vi "Control Panel.vi"(8 "error in (no error)":errorcluster, 11 "Fake Pulse Generator in":refnum<class "Pulse Generator.lvclass">) -> (0 "error out":errorcluster, 3 "Fake Pulse Generator out":refnum<class "Pulse Generator.lvclass">)   [LabVIEW 2017, in "Pulse Generator.lvclass"]
uses:
  Pulse Generator.lvclass
  Pulse Generator.lvclass/Pulse Generator.ctl
  Utility Classes/Scannable/Scannable.lvclass
panel:
  in  "Ch1/Ch2 Toggle":bool
  in  "Width/Duty\nUP/DOWN Ch2":bool
  in  "Width/Duty\nUP/DOWN Ch1":bool
  in  "Clear Error":bool
  out "Ready when \nblinking":bool
  in  "Copy actual to set":bool
  out "Pulse Mode":enum16{"Pulses", "Pattern"}(ring)
  out "Arming (Trigger) Source":T1(ring)
  in  "Populate fields with member data":bool
  out "Strobe Pattern":string
  in  "Strobe Pattern Set":string
  out "StrobeDataBuffer":digitalwaveform(graph)
  in  "Enable/disable":bool
  in  "Modes (changes immediately)":T2(radio)
  in  "BitPeriodSet":dbl[unit]
  out "BitPeriod":dbl[unit]
  out "Ch2Pattern":string
  in  "Ch2Pattern Set":string
  out "Ch1Pattern":string
  in  "Set Patterns":bool
  in  "Ch1Pattern Set":string
  in  "Ch2Duty (%) Set":dbl=10.0
  in  "Ch1Duty (%) Set":dbl=10.0
  in  "Ch1Delay Set":dbl[unit]
  in  "Ch2Delay Set":dbl[unit]
  in  "stop":bool
  out "Ch1DataBuffer":digitalwaveform(graph)
  out "Ch2DataBuffer":digitalwaveform(graph)
  in  "Ch2 Sync":bool
  in  "Ch1 Sync":bool
  in  "Ch2 Toggle":bool
  in  "Ch1 NOT Toggle":bool
  in  "Ch1 Toggle":bool
  in  "Ch2 NOT Toggle":bool
  in  "OverallPeriodSet":dbl[unit]
  in  "Ch2WidthSet":dbl[unit]=1e-09
  in  "Ch1WidthSet":dbl[unit]=1e-09
  in  "Ch2LowSet":dbl[unit]
  in  "Ch2HighSet":dbl[unit]
  in  "Ch1LowSet":dbl[unit]
  in  "Ch1HighSet":dbl[unit]
  in  "OverallFreqSet":dbl[unit]
  in  "Read to Control":bool
  in  "Set":bool
  out "Ch2Duty (%)":dbl
  out "Ch1Duty (%)":dbl
  out "Ch1Delay":dbl[unit]
  out "Ch2Delay":dbl[unit]
  out "Ch1Low":dbl[unit]
  out "Ch1High":dbl[unit]
  out "Ch2Width":dbl[unit]
  out "Ch1Width":dbl[unit]
  out "OverallPeriod":dbl[unit]
  out "Ch2Low":dbl[unit]
  out "Ch2High":dbl[unit]
  in  "Read":bool
  out "OverallFreq":dbl[unit]
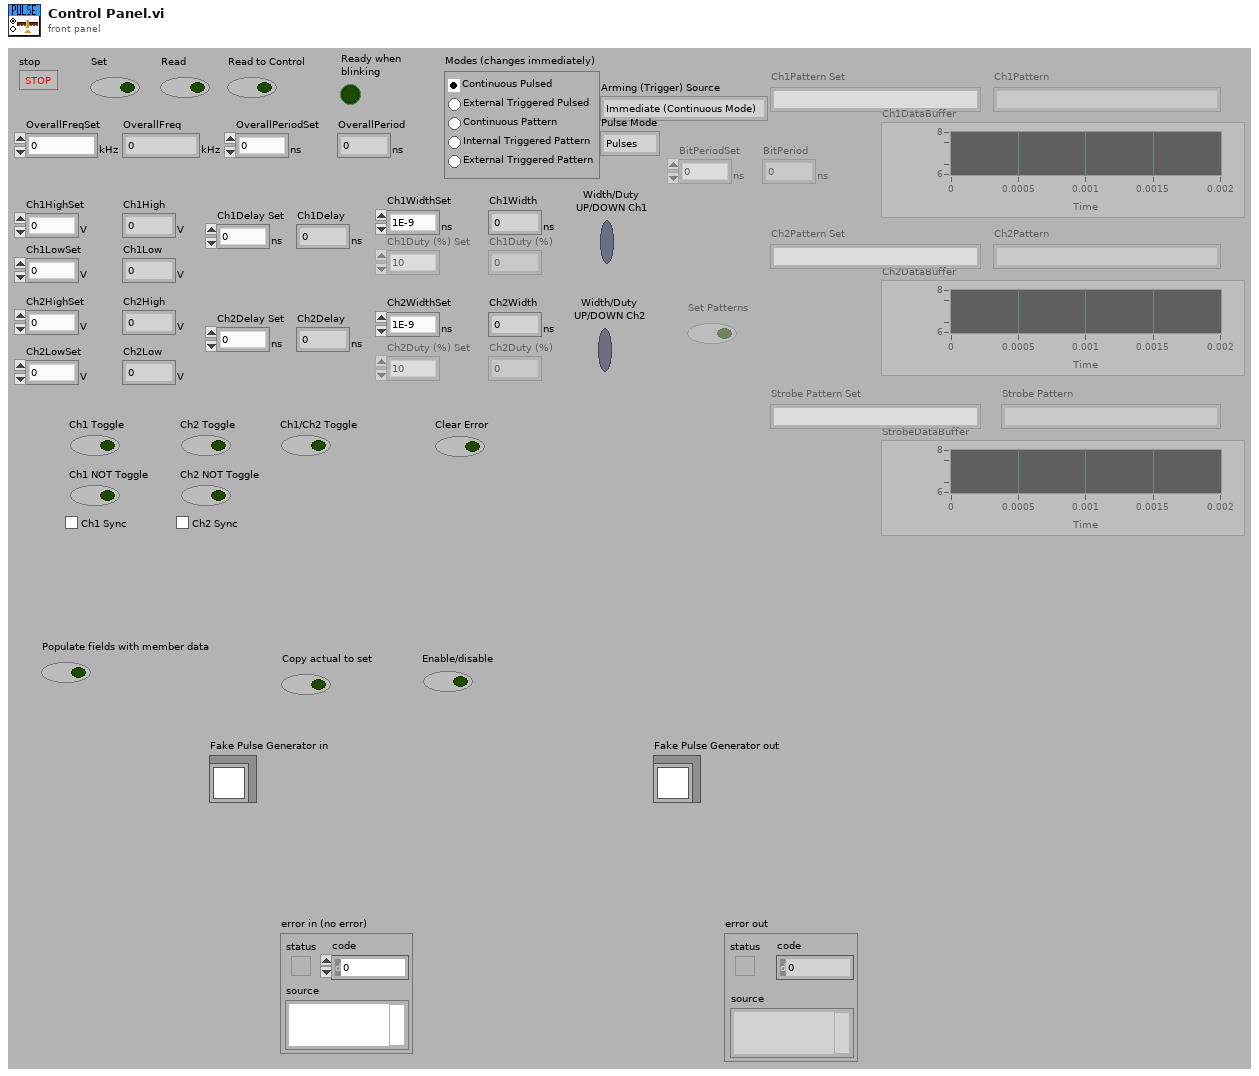
[diagram p1: front panel]
types:
  T1 = enum16{"Immediate (Continuous Mode)", "Internal PLL", "External", "Manual"}
  T2 = enum32{"Continuous Pulsed", "Continuous Pattern", "Internal Triggered Pattern", "External Triggered Pulsed", "External Triggered Pattern", "Other"}
  T3 = enum16{"Internal Oscillator", "Internal PLL", "External Clock "}
  T4 = enum16{"Internal Oscillator", "Internal PLL", "Clock Input"}
  T5 = enum16{"Channel All ", "Channel 1", "Channel 2", "Channel 3", "Channels Combined"}
  T6 = cluster{"1 High":dbl[unit], "1 Low":dbl[unit], "2 High":dbl[unit], "2 Low":dbl[unit]}
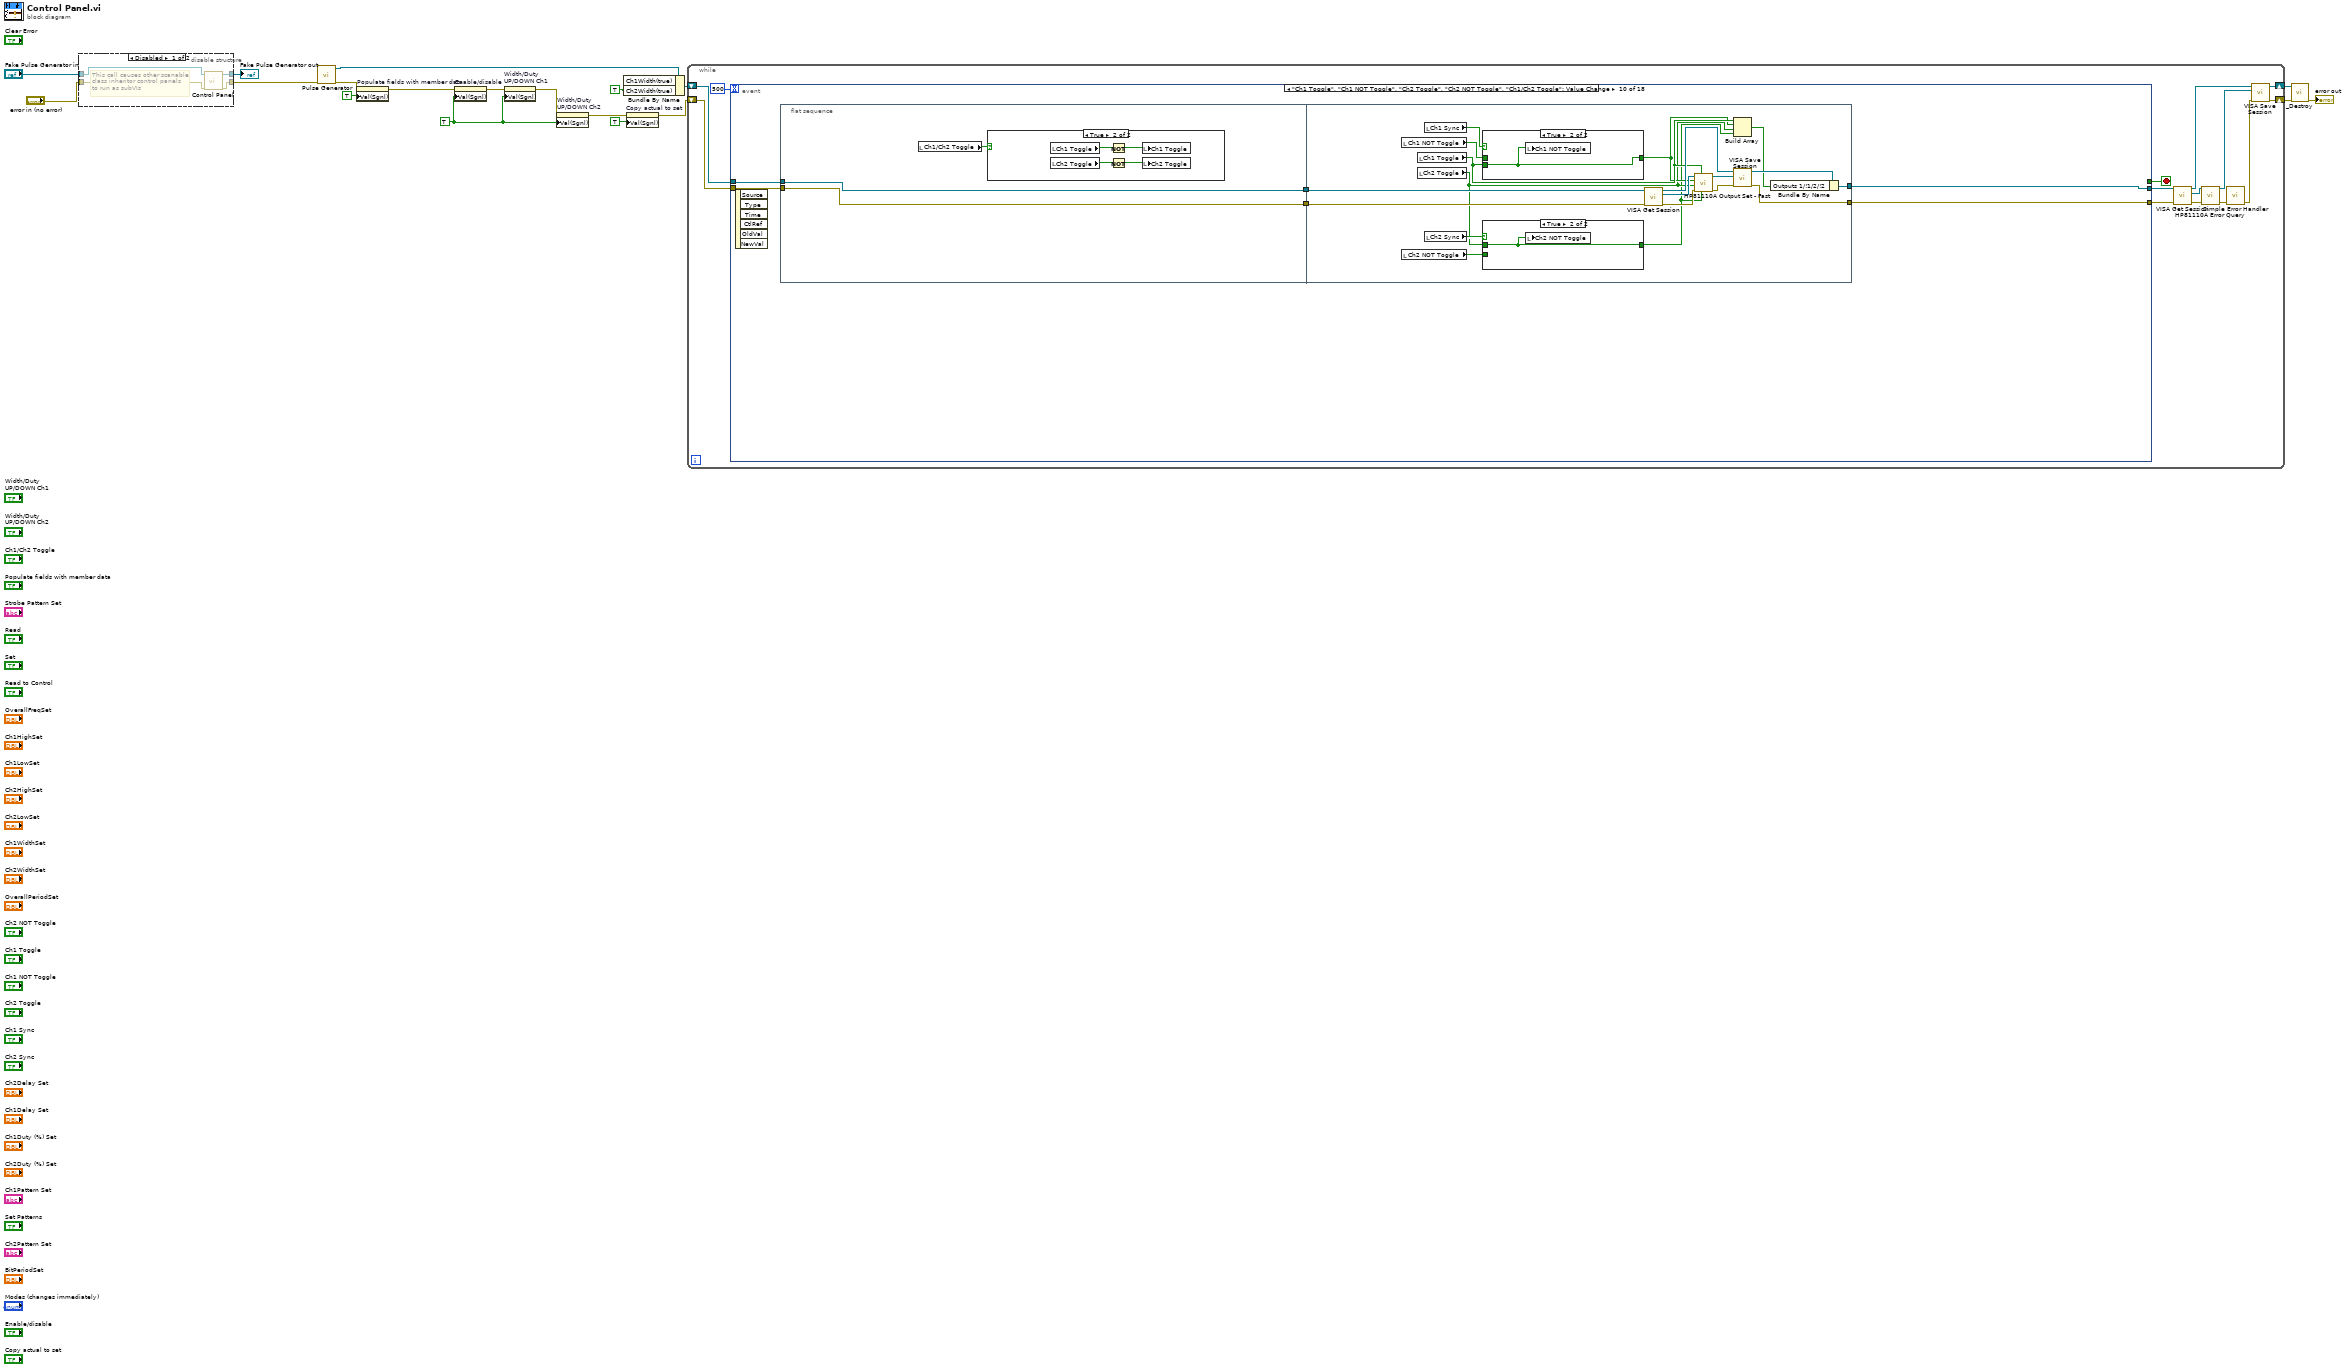
[diagram p0: block diagram]
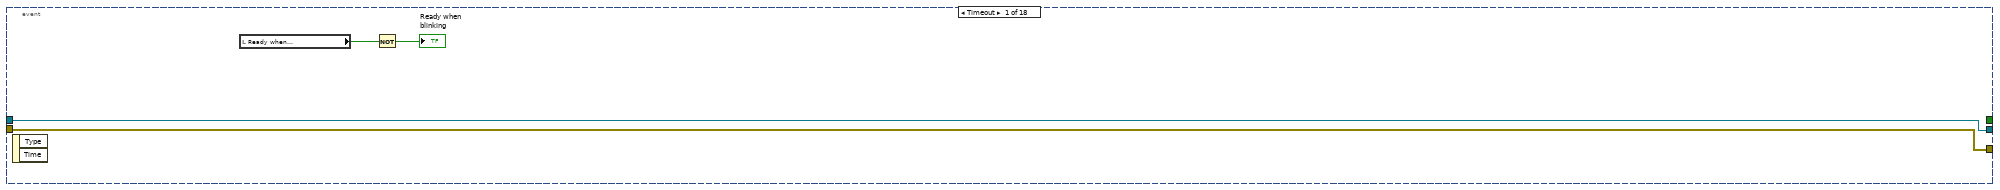
[diagram p3: hidden frame]
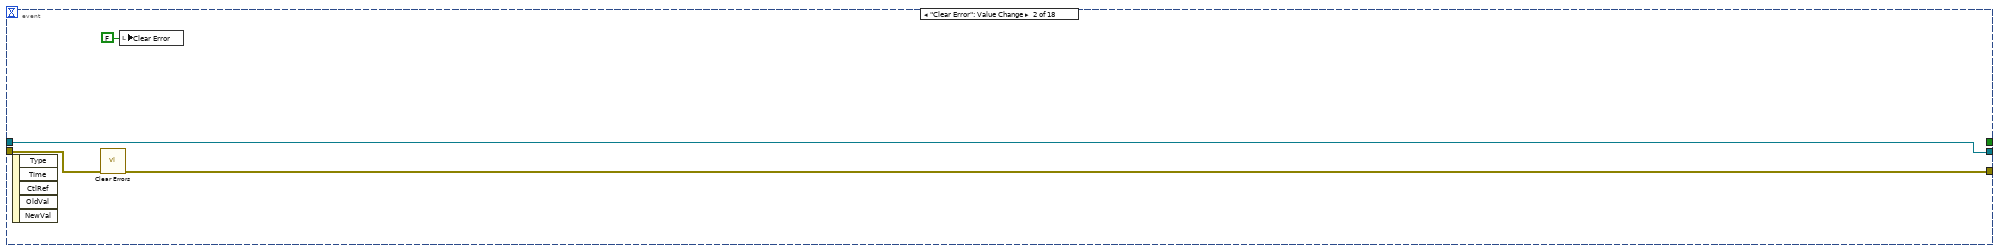
[diagram p4: hidden frame]
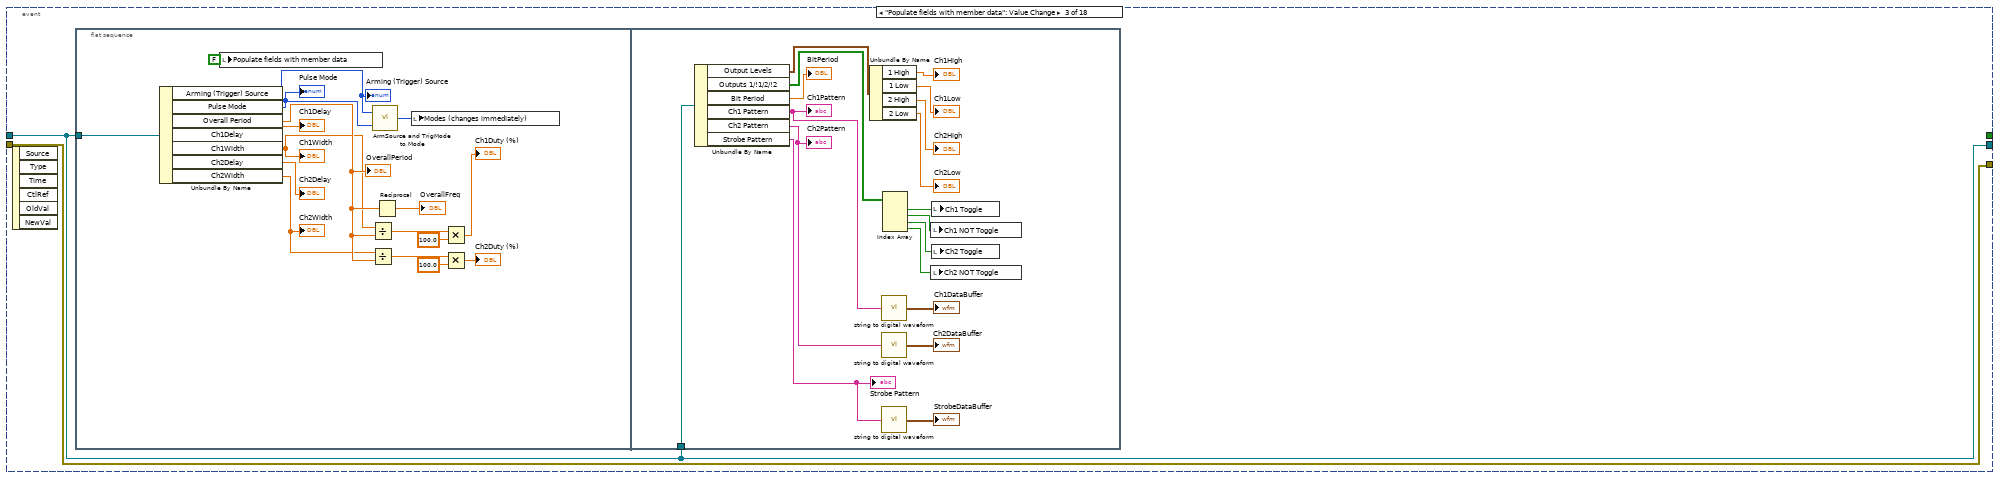
[diagram p5: hidden frame]
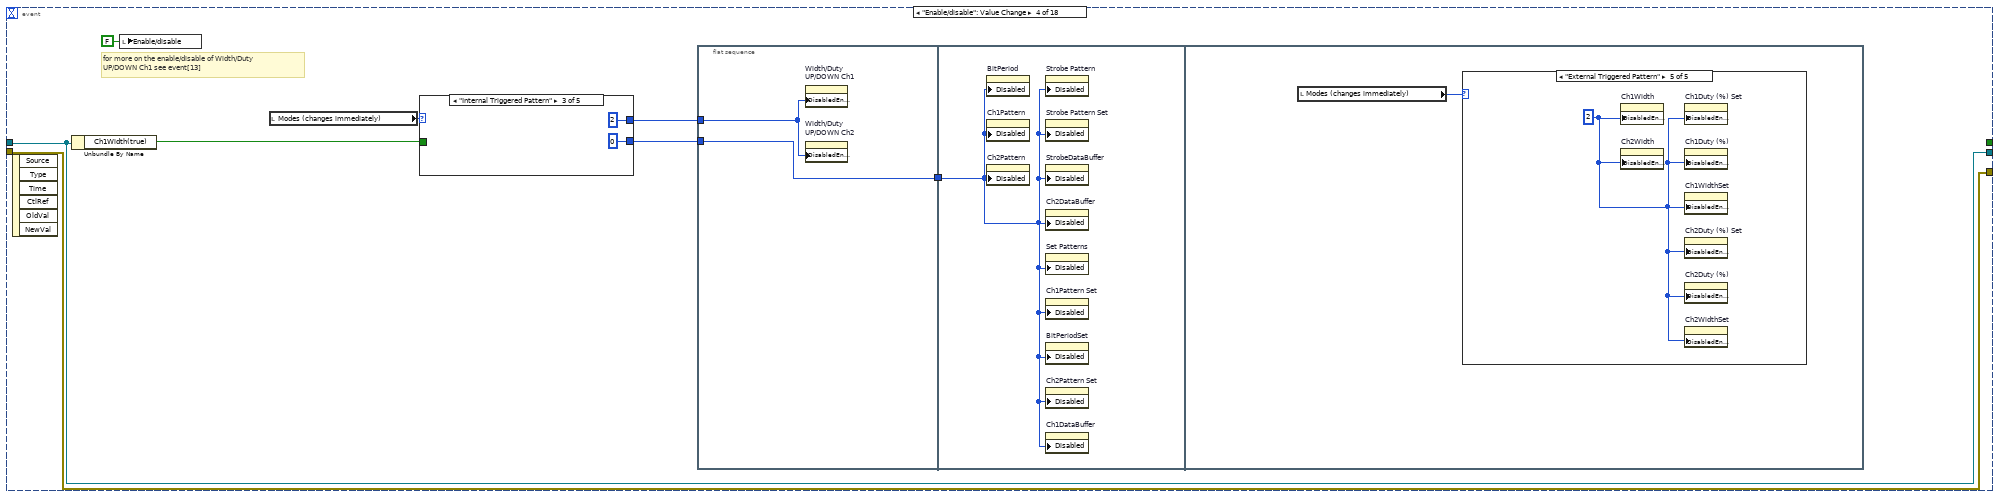
[diagram p6: hidden frame]
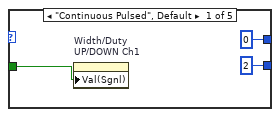
[diagram p7: hidden frame]
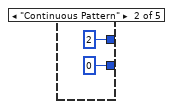
[diagram p8: hidden frame]
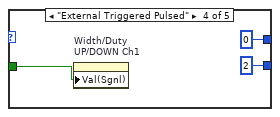
[diagram p9: hidden frame]
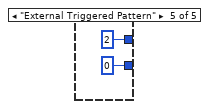
[diagram p10: hidden frame]
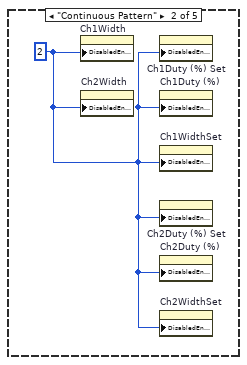
[diagram p12: hidden frame]
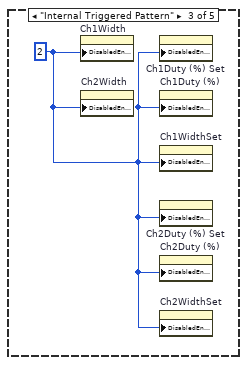
[diagram p13: hidden frame]
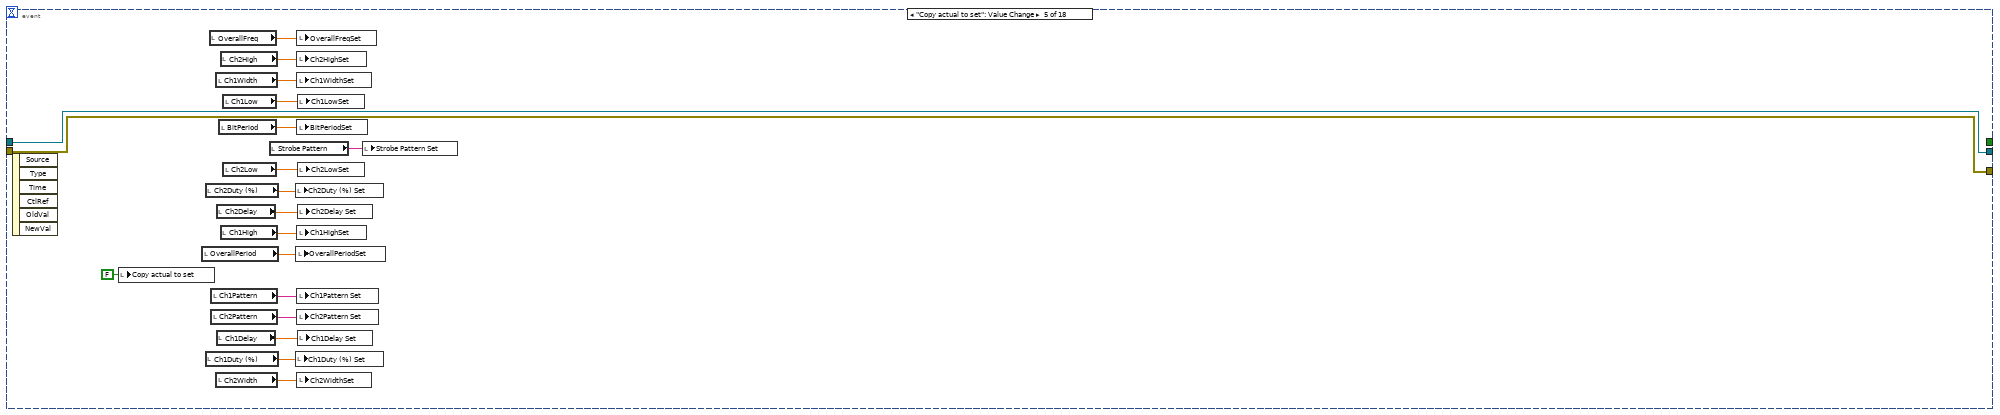
[diagram p15: hidden frame]
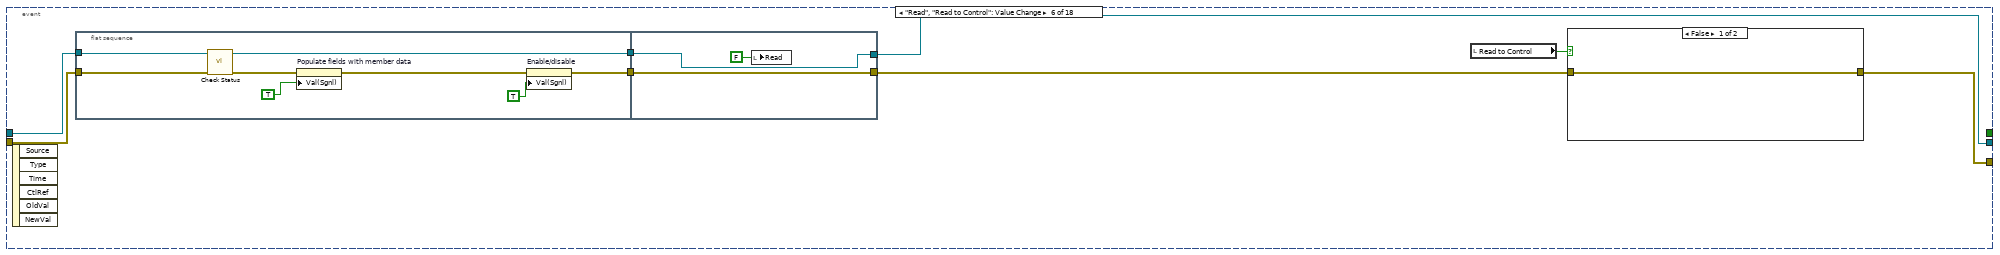
[diagram p16: hidden frame]
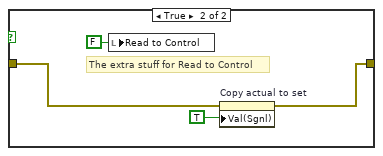
[diagram p17: hidden frame]
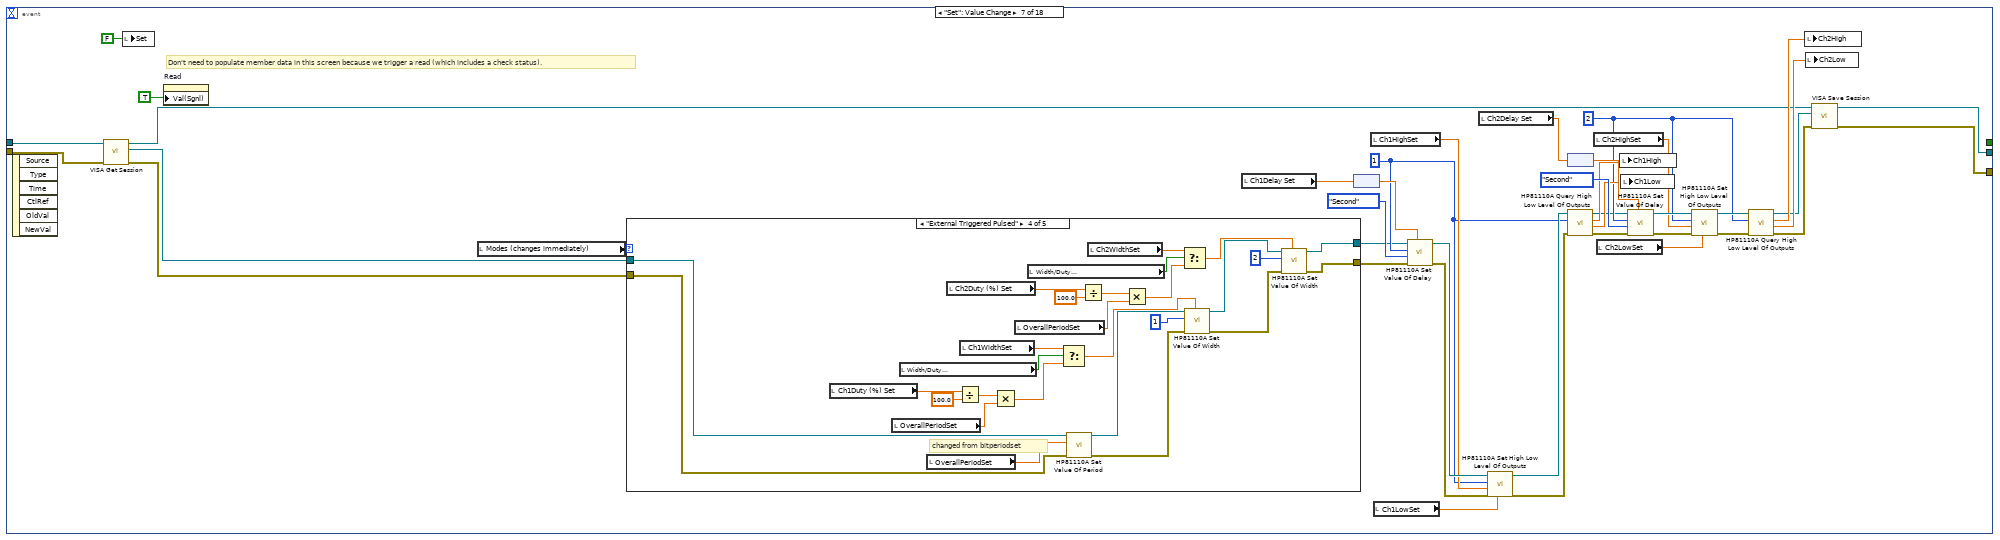
[diagram p18: hidden frame]
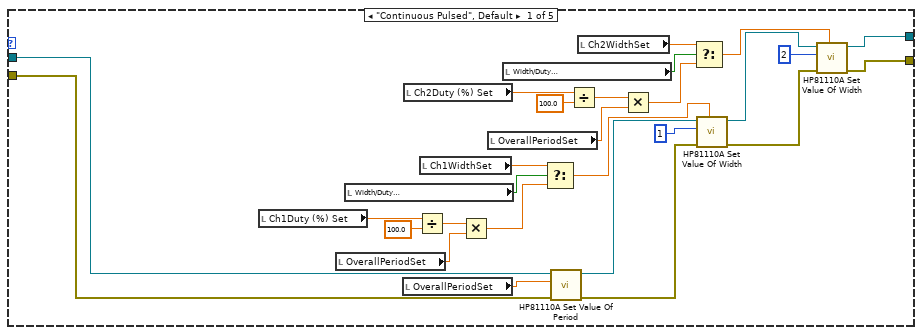
[diagram p19: hidden frame]
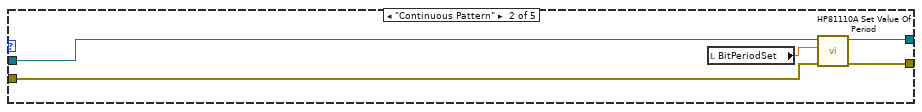
[diagram p20: hidden frame]
diagram:
  w1 = TRUE
  w4 = TRUE ("Value (Signaling)")
  n1 = disable-structure shown="Disabled" {
    disable-tunnel: [w23 w25] -> w19
    disable-tunnel: "error in (no error)" -> [w22 w24]
    disable-tunnel: "Fake Pulse Generator in" -> [w21 w25]
    disable-tunnel: [w20 w24] -> w11
    frame Disabled {
      # "This call causes other scanable\nclass inheritor control panels\nto run as subVIs"
      n2 = call-parent "Control Panel.vi"("error in (no error)"=w22, "Instrument in"=w21) -> ("error out"=w20:errorcluster, "Instrument out"=w23:refnum<class "Pulse Generator.lvclass">)  [unwired: 8 out]
    }
    frame Enabled {
    }
  }
  "Fake Pulse Generator out" <- w19
  n3 = call "Pulse Generator.vi"("error in (no error)"=w11) -> ("error out"=w12:errorcluster, "Pulse Generator out"=w3:refnum<class "Pulse Generator.lvclass">)  [unwired: 9 out]
  n4 = property on="Populate fields with member data" class="Bool (strict)"(error in=w12, "Val(Sgnl)"=TRUE ("Value (Signaling)")) -> (error out=w9:errorcluster)  [unwired: 1 in, 1 out]
  n5 = property on="Enable/disable" class="Bool (strict)"(error in=w9, "Val(Sgnl)"=w4) -> (error out=w7:errorcluster)  [unwired: 1 in, 1 out]
  n6 = property on="Width/Duty\nUP/DOWN Ch1" class="Bool (strict)"(error in=w7, "Val(Sgnl)"=w4) -> (error out=w5:errorcluster)  [unwired: 1 in, 1 out]
  n7 = property on="Width/Duty\nUP/DOWN Ch2" class="Bool (strict)"(error in=w5, "Val(Sgnl)"=w4) -> (error out=w6:errorcluster)  [unwired: 1 in, 1 out]
  n8 = Bundle By Name(cluster=w3, "Ch1Width(true)"=w1, "Ch2Width(true)"=w1) -> (w2:refnum<class "Pulse Generator.lvclass">)
  n9 = property on="Copy actual to set" class="Bool (strict)"(error in=w6, "Val(Sgnl)"=TRUE ("Value (Signaling)")) -> (error out=w8:errorcluster)  [unwired: 1 in, 1 out]
  n10 = while {
    shift-right: [w32] -> w16
    shift-left: w2 -> [w37]
    shift-right: [w27] -> w15
    shift-left: w8 -> [w36]
    stop <- w39 stop-if-true
    n11 = event shown="[9] \"Ch1 Toggle\", \"Ch1 NOT Toggle\", \"Ch2 Toggle\", \"Ch2 NOT Toggle\", \"Ch1/Ch2 Toggle\": Value Change" {
      selector: _ -> [_ _ _ _ _ _ _ _ _ _ _ _ _ _ _ _ _ _]
      dyn-events: _ -> [_ _ _ _ _ _ _ _ _ _ _ _ _ _ _ _ _ _]
      timeout: 500 -> [_ _ _ _ _ _ _ _ _ _ _ _ _ _ _ _ _ _]
      tunnel: [_ _ _ _ _ _ _ _ _ _ _ _ "stop" _ _ _ _ _] -> w39
      tunnel: w36 -> [w42 w47 w49 w91 w113 w138 w161 w273 w311 w327 w362 w385 w398 w418 w420 w430 w440 w446]
      tunnel: [w42 w45 w49 w91 w113 w134 w157 w269 w305 w326 w362 w385 w398 w418 w420 w430 w440 w446] -> w30
      tunnel: w37 -> [w43 w46 w48 w86 w114 w137 w163 w275 w312 w328 w363 w386 w397 w405 w419 w429 w439 w447]
      tunnel: [w43 w46 w48 w86 w114 w136 w158 w270 w307 w325 w363 w386 w397 w404 w419 w429 w439 w447] -> w31
      event Timeout {
        n12 = event-data() -> ()  [unwired: 3 out]
        n13 = local read "Ready when \nblinking"() -> (w41:bool)
        n14 = Not(x=w41) -> (.not. x?=→"Ready when \nblinking":bool)
      }
      event "Clear Error": Value Change {
        n15 = event-data() -> ()  [unwired: 6 out]
        n16 = call <vilib>:"Clear Errors.vi"("error in (no error)"=w47) -> ("error out"=w45:errorcluster)  [unwired: 5 in, 1 out]
        n17 = local write "Clear Error"(FALSE ("Clear Error")) -> ()
      }
      event "Populate fields with member data": Value Change {
        n18 = event-data() -> ()  [unwired: 7 out]
        n19 = flat-sequence {
          tunnel: w48 -> [w56]
          tunnel: w48 -> [w67]
          frame #0 {
            n20 = Unbundle By Name(w56) -> ("Arming (Trigger) Source"=w59:u16, "Pulse Mode"=w58:u16, "Overall Period"=w62:dbl[unit], "Ch1Delay"=→"Ch1Delay":dbl[unit], "Ch1Width"=w61:dbl[unit], "Ch2Delay"=→"Ch2Delay":dbl[unit], "Ch2Width"=w60:dbl[unit])
            "OverallPeriod" <- w62
            "Ch1Width" <- w61
            "Ch2Width" <- w60
            "Arming (Trigger) Source" <- w59
            "Pulse Mode" <- w58
            n21 = local write "Populate fields with member data"(FALSE ("Populate fields with member data")) -> ()
            n22 = Divide(x=w61, y=w62) -> (x/y=w53:dbl)
            n23 = Divide(x=w60, y=w62) -> (x/y=w51:dbl)
            n24 = call "ArmSource and TrigMode to Mode.vi"("Pulse Mode"=w58, "Arming (Trigger) Source (0:Internal PLL)"=w59) -> ("Modes (changes immediately)"=w57:T2)
            n25 = Reciprocal(x=w62) -> (1/x=→"OverallFreq":dbl[unit])
            n26 = local write "Modes (changes immediately)"(w57) -> ()
            n27 = Multiply(x=w53, y=100.0) -> (x*y=→"Ch1Duty (%)":dbl)
            n28 = Multiply(x=w51, y=100.0) -> (x*y=→"Ch2Duty (%)":dbl)
          }
          frame #1 {
            n29 = Unbundle By Name(w67) -> ("Output Levels"=w79:T6, "Outputs 1/!1/2/!2"=w80:bool[], "Bit Period"=→"BitPeriod":dbl[unit], "Ch1 Pattern"=w82:string, "Ch2 Pattern"=w83:string, "Strobe Pattern"=w84:string)
            "Ch1Pattern" <- w82
            "Ch2Pattern" <- w83
            "Strobe Pattern" <- w84
            n30 = Unbundle By Name(w79) -> ("1 High"=→"Ch1High":dbl[unit], "1 Low"=→"Ch1Low":dbl[unit], "2 High"=→"Ch2High":dbl[unit], "2 Low"=→"Ch2Low":dbl[unit])
            n31 = call "string to digital waveform.vi"("String"=w82) -> ("digital waveform"=→"Ch1DataBuffer":digitalwaveform)
            n32 = call "string to digital waveform.vi"("String"=w83) -> ("digital waveform"=→"Ch2DataBuffer":digitalwaveform)
            n33 = call "string to digital waveform.vi"("String"=w84) -> ("digital waveform"=→"StrobeDataBuffer":digitalwaveform)
            n34 = Index Array(array=w80) -> (element #1=w75:bool, element #2=w76:bool, element #3=w77:bool, element #4=w78:bool)  [unwired: 4 in]
            n35 = local write "Ch1 NOT Toggle"(w76) -> ()
            n36 = local write "Ch2 NOT Toggle"(w78) -> ()
            n37 = local write "Ch1 Toggle"(w75) -> ()
            n38 = local write "Ch2 Toggle"(w77) -> ()
          }
        }
      }
      event "Enable/disable": Value Change {
        # "for more on the enable/disable of Width/Duty\nUP/DOWN Ch1 see event[13]"
        n39 = event-data() -> ()  [unwired: 7 out]
        n40 = Unbundle By Name(w86) -> ("Ch1Width(true)"=w85:bool)
        n41 = local write "Enable/disable"(FALSE ("Enable/disable")) -> ()
        n42 = local read "Modes (changes immediately)"() -> (w89:T2)
        n43 = case shown="\"Internal Triggered Pattern\"" w89 {
          tunnel: [2 0 0 2 0] -> w87
          tunnel: [0 2 2 0 2] -> w88
          tunnel: w85 -> [w93 _ _ w100 _]
          frame "Continuous Pulsed", Default {
            n44 = property on="Width/Duty\nUP/DOWN Ch1" class="Bool (strict)"("Val(Sgnl)"=w93) -> ()  [unwired: 2 in, 2 out]
          }
          frame "Continuous Pattern" {
          }
          frame "Internal Triggered Pattern" {
          }
          frame "External Triggered Pulsed" {
            n45 = property on="Width/Duty\nUP/DOWN Ch1" class="Bool (strict)"("Val(Sgnl)"=w100) -> ()  [unwired: 2 in, 2 out]
          }
          frame "External Triggered Pattern" {
          }
        }
        n46 = flat-sequence {
          tunnel: [w106] -> w90
          tunnel: w88 -> [w105]
          tunnel: w87 -> [w106]
          tunnel: w90 -> [w107]
          frame #0 {
            n47 = property on="Width/Duty\nUP/DOWN Ch1" class="Bool (strict)"("DisabledEnum"=w105) -> ()  [unwired: 2 in, 2 out]
            n48 = property on="Width/Duty\nUP/DOWN Ch2" class="Bool (strict)"("DisabledEnum"=w105) -> ()  [unwired: 2 in, 2 out]
          }
          frame #1 {
            n49 = property on="BitPeriod" class="DigNum (strict)"("Disabled"=w107) -> ()  [unwired: 2 in, 2 out]
            n50 = property on="Ch1Pattern" class="Str"("Disabled"=w107) -> ()  [unwired: 2 in, 2 out]
            n51 = property on="Ch2Pattern" class="Str"("Disabled"=w107) -> ()  [unwired: 2 in, 2 out]
            n52 = property on="Strobe Pattern" class="Str"("Disabled"=w107) -> ()  [unwired: 2 in, 2 out]
            n53 = property on="Strobe Pattern Set" class="Str"("Disabled"=w107) -> ()  [unwired: 2 in, 2 out]
            n54 = property on="StrobeDataBuffer" class="DigitalGraph (strict)"("Disabled"=w107) -> ()  [unwired: 2 in, 2 out]
            n55 = property on="Ch2DataBuffer" class="DigitalGraph (strict)"("Disabled"=w107) -> ()  [unwired: 2 in, 2 out]
            n56 = property on="Set Patterns" class="Bool (strict)"("Disabled"=w107) -> ()  [unwired: 2 in, 2 out]
            n57 = property on="Ch1Pattern Set" class="Str"("Disabled"=w107) -> ()  [unwired: 2 in, 2 out]
            n58 = property on="BitPeriodSet" class="DigNum (strict)"("Disabled"=w107) -> ()  [unwired: 2 in, 2 out]
            n59 = property on="Ch2Pattern Set" class="Str"("Disabled"=w107) -> ()  [unwired: 2 in, 2 out]
            n60 = property on="Ch1DataBuffer" class="DigitalGraph (strict)"("Disabled"=w107) -> ()  [unwired: 2 in, 2 out]
          }
          frame #2 {
            n61 = local read "Modes (changes immediately)"() -> (w108:T2)
            n62 = case shown="\"External Triggered Pattern\"" w108 {
              frame "Continuous Pulsed", Default {
              }
              frame "Continuous Pattern" {
                w109 = 2
                n63 = property on="Ch1Width" class="DigNum (strict)"("DisabledEnum"=w109) -> ()  [unwired: 2 in, 2 out]
                n64 = property on="Ch2Width" class="DigNum (strict)"("DisabledEnum"=w109) -> ()  [unwired: 2 in, 2 out]
                n65 = property on="Ch1Duty (%) Set" class="DigNum (strict)"("DisabledEnum"=w109) -> ()  [unwired: 2 in, 2 out]
                n66 = property on="Ch1Duty (%)" class="DigNum (strict)"("DisabledEnum"=w109) -> ()  [unwired: 2 in, 2 out]
                n67 = property on="Ch1WidthSet" class="DigNum (strict)"("DisabledEnum"=w109) -> ()  [unwired: 2 in, 2 out]
                n68 = property on="Ch2Duty (%) Set" class="DigNum (strict)"("DisabledEnum"=w109) -> ()  [unwired: 2 in, 2 out]
                n69 = property on="Ch2Duty (%)" class="DigNum (strict)"("DisabledEnum"=w109) -> ()  [unwired: 2 in, 2 out]
                n70 = property on="Ch2WidthSet" class="DigNum (strict)"("DisabledEnum"=w109) -> ()  [unwired: 2 in, 2 out]
              }
              frame "Internal Triggered Pattern" {
                w110 = 2
                n71 = property on="Ch1Width" class="DigNum (strict)"("DisabledEnum"=w110) -> ()  [unwired: 2 in, 2 out]
                n72 = property on="Ch2Width" class="DigNum (strict)"("DisabledEnum"=w110) -> ()  [unwired: 2 in, 2 out]
                n73 = property on="Ch1Duty (%) Set" class="DigNum (strict)"("DisabledEnum"=w110) -> ()  [unwired: 2 in, 2 out]
                n74 = property on="Ch1Duty (%)" class="DigNum (strict)"("DisabledEnum"=w110) -> ()  [unwired: 2 in, 2 out]
                n75 = property on="Ch1WidthSet" class="DigNum (strict)"("DisabledEnum"=w110) -> ()  [unwired: 2 in, 2 out]
                n76 = property on="Ch2Duty (%) Set" class="DigNum (strict)"("DisabledEnum"=w110) -> ()  [unwired: 2 in, 2 out]
                n77 = property on="Ch2Duty (%)" class="DigNum (strict)"("DisabledEnum"=w110) -> ()  [unwired: 2 in, 2 out]
                n78 = property on="Ch2WidthSet" class="DigNum (strict)"("DisabledEnum"=w110) -> ()  [unwired: 2 in, 2 out]
              }
              frame "External Triggered Pulsed" {
              }
              frame "External Triggered Pattern" {
                w111 = 2
                n79 = property on="Ch1Width" class="DigNum (strict)"("DisabledEnum"=w111) -> ()  [unwired: 2 in, 2 out]
                n80 = property on="Ch2Width" class="DigNum (strict)"("DisabledEnum"=w111) -> ()  [unwired: 2 in, 2 out]
                n81 = property on="Ch1Duty (%) Set" class="DigNum (strict)"("DisabledEnum"=w111) -> ()  [unwired: 2 in, 2 out]
                n82 = property on="Ch1Duty (%)" class="DigNum (strict)"("DisabledEnum"=w111) -> ()  [unwired: 2 in, 2 out]
                n83 = property on="Ch1WidthSet" class="DigNum (strict)"("DisabledEnum"=w111) -> ()  [unwired: 2 in, 2 out]
                n84 = property on="Ch2Duty (%) Set" class="DigNum (strict)"("DisabledEnum"=w111) -> ()  [unwired: 2 in, 2 out]
                n85 = property on="Ch2Duty (%)" class="DigNum (strict)"("DisabledEnum"=w111) -> ()  [unwired: 2 in, 2 out]
                n86 = property on="Ch2WidthSet" class="DigNum (strict)"("DisabledEnum"=w111) -> ()  [unwired: 2 in, 2 out]
              }
            }
          }
        }
      }
      event "Copy actual to set": Value Change {
        n87 = event-data() -> ()  [unwired: 7 out]
        n88 = local write "Copy actual to set"(FALSE ("Copy actual to set")) -> ()
        n89 = local read "OverallPeriod"() -> (w129:dbl[unit])
        n90 = local read "Ch2Duty (%)"() -> (w121:dbl)
        n91 = local read "Ch1Duty (%)"() -> (w125:dbl)
        n92 = local read "OverallFreq"() -> (w130:dbl[unit])
        n93 = local read "Ch1Pattern"() -> (w118:string)
        n94 = local read "Ch2Pattern"() -> (w117:string)
        n95 = local read "Ch1Width"() -> (w126:dbl[unit])
        n96 = local read "Ch2Width"() -> (w122:dbl[unit])
        n97 = local read "Ch2Delay"() -> (w120:dbl[unit])
        n98 = local read "Ch1Delay"() -> (w124:dbl[unit])
        n99 = local read "BitPeriod"() -> (w116:dbl[unit])
        n100 = local read "Ch2High"() -> (w119:dbl[unit])
        n101 = local read "Ch1High"() -> (w128:dbl[unit])
        n102 = local read "Ch1Low"() -> (w127:dbl[unit])
        n103 = local read "Ch2Low"() -> (w123:dbl[unit])
        n104 = local read "Strobe Pattern"() -> (w112:string)
        n105 = local write "Ch2Duty (%) Set"(w121) -> ()
        n106 = local write "Ch1Duty (%) Set"(w125) -> ()
        n107 = local write "OverallPeriodSet"(w129) -> ()
        n108 = local write "OverallFreqSet"(w130) -> ()
        n109 = local write "Ch2HighSet"(w119) -> ()
        n110 = local write "Ch1WidthSet"(w126) -> ()
        n111 = local write "BitPeriodSet"(w116) -> ()
        n112 = local write "Ch1HighSet"(w128) -> ()
        n113 = local write "Ch1Pattern Set"(w118) -> ()
        n114 = local write "Ch2Pattern Set"(w117) -> ()
        n115 = local write "Ch2WidthSet"(w122) -> ()
        n116 = local write "Ch1LowSet"(w127) -> ()
        n117 = local write "Ch2LowSet"(w123) -> ()
        n118 = local write "Ch2Delay Set"(w120) -> ()
        n119 = local write "Ch1Delay Set"(w124) -> ()
        n120 = local write "Strobe Pattern Set"(w112) -> ()
      }
      event "Read", "Read to Control": Value Change {
        n121 = event-data() -> ()  [unwired: 7 out]
        n122 = flat-sequence {
          tunnel: w138 -> [w146]
          tunnel: w137 -> [w145]
          tunnel: [w144] -> w132
          tunnel: [w143] -> w131
          tunnel: [w148] -> w135
          tunnel: [w149] -> w136
          tunnel: w132 -> [w149]
          tunnel: w131 -> [w148]
          frame #0 {
            n123 = call-dynamic "Check Status.vi"("error in (no error)"=w146, "Pulse Generator in"=w145) -> ("error out"=w140:errorcluster, "Pulse Generator out"=w144:refnum<class "Pulse Generator.lvclass">)  [unwired: 8 out]
            n124 = property on="Populate fields with member data" class="Bool (strict)"(error in=w140, "Val(Sgnl)"=TRUE ("Value (Signaling)")) -> (error out=w139:errorcluster)  [unwired: 1 in, 1 out]
            n125 = property on="Enable/disable" class="Bool (strict)"(error in=w139, "Val(Sgnl)"=TRUE ("Value (Signaling)")) -> (error out=w143:errorcluster)  [unwired: 1 in, 1 out]
          }
          frame #1 {
            n126 = local write "Read"(FALSE) -> ()
          }
        }
        n127 = local read "Read to Control"() -> (w133:bool)
        n128 = case shown="False" w133 {
          tunnel: w135 -> [w150 w152]
          tunnel: [w150 w151] -> w134
          frame False {
          }
          frame True {
            # "The extra stuff for Read to Control"
            n129 = local write "Read to Control"(FALSE) -> ()
            n130 = property on="Copy actual to set" class="Bool (strict)"(error in=w152, "Val(Sgnl)"=TRUE ("Value (Signaling)")) -> (error out=w151:errorcluster)  [unwired: 1 in, 1 out]
          }
        }
      }
      event "Set": Value Change {
        w169 = 1
        w174 = 2
        # "Don't need to populate member data in this screen because we trigger a read (which includes a check status)."
        n131 = event-data() -> ()  [unwired: 7 out]
        n132 = call-dynamic "VISA Get Session.vi"("error in (no error)"=w161, "Instrument.lvclass in"=w163) -> ("error out"=w160:errorcluster, "VISA Resource Name"=w162:refnum<visa-resource-name>, "Instrument.lvclass out"=w159:refnum<class "Pulse Generator.lvclass">)  [unwired: 7 out]
        n133 = local write "Set"(FALSE) -> ()
        n134 = property on="Read" class="Bool (strict)"("Val(Sgnl)"=TRUE ("Value (Signaling)")) -> ()  [unwired: 2 in, 2 out]
        n135 = local read "Modes (changes immediately)"() -> (w166:T2)
        n136 = case shown="\"External Triggered Pulsed\"" w166 {
          tunnel: w162 -> [w216 w225 w230 w257 w265]
          tunnel: w160 -> [w215 w223 w228 w254 w263]
          tunnel: [w212 w224 w229 w255 w264] -> w165
          tunnel: [w211 w222 w227 w252 w263] -> w164
          frame "Continuous Pulsed", Default {
            n137 = local read "Ch1Duty (%) Set"() -> (w207:dbl)
            n138 = local read "OverallPeriodSet"() -> (w205:dbl[unit])
            n139 = local read "Width/Duty\nUP/DOWN Ch1"() -> (w210:bool)
            n140 = local read "OverallPeriodSet"() -> (w221:dbl[unit])
            n141 = local read "Ch2Duty (%) Set"() -> (w201:dbl)
            n142 = Divide(x=w207, y=100.0) -> (x/y=w206:dbl)
            n143 = local read "Ch1WidthSet"() -> (w209:dbl[unit])
            n144 = Multiply(x=w206, y=w205) -> (x*y=w204:dbl[unit])
            n145 = local read "OverallPeriodSet"() -> (w203:dbl[unit])
            n146 = local read "Width/Duty\nUP/DOWN Ch2"() -> (w198:bool)
            n147 = Select(t=w209, s=w210, f=w204) -> (s? t:f=w195:dbl[unit])
            n148 = call "HP81110A Set Value Of Period.vi"("error in (no error)"=w215, "Period Value"=w221, "VISA session"=w216) -> ("error out"=w213:errorcluster, "dup VISA session"=w214:refnum<visa-resource-name>)  [unwired: 7 out]
            n149 = Divide(x=w201, y=100.0) -> (x/y=w202:dbl)
            n150 = local read "Ch2WidthSet"() -> (w197:dbl[unit])
            n151 = Multiply(x=w202, y=w203) -> (x*y=w199:dbl[unit])
            n152 = Select(t=w197, s=w198, f=w199) -> (s? t:f=w196:dbl[unit])
            n153 = call "HP81110A Set Value Of Width.vi"("Width Value (100.0E-9)"=w195, "error in (no error)"=w213, "Channel (1:Channel 1)"=1, "VISA session"=w214) -> ("error out"=w220:errorcluster, "dup VISA session"=w219:refnum<visa-resource-name>)  [unwired: 1 in, 5 out]
            n154 = call "HP81110A Set Value Of Width.vi"("Width Value (100.0E-9)"=w196, "error in (no error)"=w220, "Channel (1:Channel 1)"=2, "VISA session"=w219) -> ("error out"=w211:errorcluster, "dup VISA session"=w212:refnum<visa-resource-name>)  [unwired: 1 in, 5 out]
          }
          frame "Continuous Pattern" {
            n155 = local read "BitPeriodSet"() -> (w226:dbl[unit])
            n156 = call "HP81110A Set Value Of Period.vi"("error in (no error)"=w223, "Period Value"=w226, "VISA session"=w225) -> ("error out"=w222:errorcluster, "dup VISA session"=w224:refnum<visa-resource-name>)  [unwired: 7 out]
          }
          frame "Internal Triggered Pattern" {
            n157 = local read "OverallPeriodSet"() -> (w232:dbl[unit])
            n158 = local read "BitPeriodSet"() -> (w231:dbl[unit])
            n159 = node(w232) -> (w233:dbl)
            n160 = call "HP81110A Set Value Of Period.vi"("error in (no error)"=w228, "Period Value"=w231, "VISA session"=w230) -> ("error out"=w235:errorcluster, "dup VISA session"=w234:refnum<visa-resource-name>)  [unwired: 7 out]
            n161 = call "HP81110A Set Arming Period.vi"("error in (no error)"=w235, "Period Value (10.0E-6 Sec)"=w233, "VISA session"=w234) -> ("error out"=w227:errorcluster, "dup VISA session"=w229:refnum<visa-resource-name>)  [unwired: 7 out]
          }
          frame "External Triggered Pulsed" {
            # "changed from bitperiodset"
            n162 = local read "Ch1Duty (%) Set"() -> (w248:dbl)
            n163 = local read "OverallPeriodSet"() -> (w246:dbl[unit])
            n164 = local read "Width/Duty\nUP/DOWN Ch1"() -> (w251:bool)
            n165 = local read "OverallPeriodSet"() -> (w258:dbl[unit])
            n166 = local read "Ch2Duty (%) Set"() -> (w242:dbl)
            n167 = Divide(x=w248, y=100.0) -> (x/y=w247:dbl)
            n168 = local read "Ch1WidthSet"() -> (w250:dbl[unit])
            n169 = Multiply(x=w247, y=w246) -> (x*y=w245:dbl[unit])
            n170 = local read "OverallPeriodSet"() -> (w244:dbl[unit])
            n171 = local read "Width/Duty\nUP/DOWN Ch2"() -> (w240:bool)
            n172 = Select(t=w250, s=w251, f=w245) -> (s? t:f=w238:dbl[unit])
            n173 = call "HP81110A Set Value Of Period.vi"("error in (no error)"=w254, "Period Value"=w258, "VISA session"=w257) -> ("error out"=w253:errorcluster, "dup VISA session"=w256:refnum<visa-resource-name>)  [unwired: 7 out]
            n174 = Divide(x=w242, y=100.0) -> (x/y=w243:dbl)
            n175 = local read "Ch2WidthSet"() -> (w239:dbl[unit])
            n176 = Multiply(x=w243, y=w244) -> (x*y=w236:dbl[unit])
            n177 = Select(t=w239, s=w240, f=w236) -> (s? t:f=w237:dbl[unit])
            n178 = call "HP81110A Set Value Of Width.vi"("Width Value (100.0E-9)"=w238, "error in (no error)"=w253, "Channel (1:Channel 1)"=1, "VISA session"=w256) -> ("error out"=w262:errorcluster, "dup VISA session"=w261:refnum<visa-resource-name>)  [unwired: 1 in, 5 out]
            n179 = call "HP81110A Set Value Of Width.vi"("Width Value (100.0E-9)"=w237, "error in (no error)"=w262, "Channel (1:Channel 1)"=2, "VISA session"=w261) -> ("error out"=w252:errorcluster, "dup VISA session"=w255:refnum<visa-resource-name>)  [unwired: 1 in, 5 out]
          }
          frame "External Triggered Pattern" {
            n180 = local read "BitPeriodSet"() -> (w266:dbl[unit])
            n181 = call "HP81110A Set Value Of Period.vi"("Period Value"=w266, "VISA session"=w265) -> ("dup VISA session"=w264:refnum<visa-resource-name>)  [unwired: 1 in, 8 out]
          }
        }
        n182 = local read "Ch1Delay Set"() -> (w192:dbl[unit])
        n183 = node(w192) -> (w191:dbl)
        n184 = local read "Ch1HighSet"() -> (w178:dbl[unit])
        n185 = local read "Ch1LowSet"() -> (w177:dbl[unit])
        n186 = call "HP81110A Set Value Of Delay.vi"("Delay Value (0.0)"=w191, "error in (no error)"=w164, "Delay Unit (0:Second)"=enum16{"Second", "Percent", "Degree", "Radians"}."Second", "Channel (1:Channel 1)"=w169, "VISA session"=w165) -> ("error out"=w182:errorcluster, "dup VISA session"=w181:refnum<visa-resource-name>)  [unwired: 5 out]
        n187 = local read "Ch2Delay Set"() -> (w190:dbl[unit])
        n188 = call "HP81110A Set High Low Level Of Outputs.vi"("Value Low (-0.5 V)"=w177, "error in (no error)"=w182, "Value High (0.5 V)"=w178, "Channel (1:Channel 1)"=w169, "VISA session"=w181) -> ("error out"=w179:errorcluster, "dup VISA session"=w180:refnum<visa-resource-name>)  [unwired: 5 out]
        n189 = node(w190) -> (w189:dbl)
        n190 = call "HP81110A Query High Low Level Of Outputs.vi"("error in (no error)"=w179, "Channel (1:Channel 1)"=w169, "VISA session"=w180) -> ("error out"=w167:errorcluster, "Value Low"=w175:dbl[unit], "Value High"=w176:dbl[unit], "dup VISA session"=w168:refnum<visa-resource-name>)  [unwired: 5 out]
        n191 = local read "Ch2HighSet"() -> (w173:dbl[unit])
        n192 = local read "Ch2LowSet"() -> (w172:dbl[unit])
        n193 = local write "Ch1High"(w176) -> ()
        n194 = local write "Ch1Low"(w175) -> ()
        n195 = call "HP81110A Set Value Of Delay.vi"("Delay Value (0.0)"=w189, "error in (no error)"=w167, "Delay Unit (0:Second)"=enum16{"Second", "Percent", "Degree", "Radians"}."Second", "Channel (1:Channel 1)"=w174, "VISA session"=w168) -> ("error out"=w184:errorcluster, "dup VISA session"=w186:refnum<visa-resource-name>)  [unwired: 5 out]
        n196 = call "HP81110A Set High Low Level Of Outputs.vi"("Value Low (-0.5 V)"=w172, "error in (no error)"=w184, "Value High (0.5 V)"=w173, "Channel (1:Channel 1)"=w174, "VISA session"=w186) -> ("error out"=w183:errorcluster, "dup VISA session"=w185:refnum<visa-resource-name>)  [unwired: 5 out]
        n197 = call "HP81110A Query High Low Level Of Outputs.vi"("error in (no error)"=w183, "Channel (1:Channel 1)"=w174, "VISA session"=w185) -> ("error out"=w155:errorcluster, "Value Low"=w170:dbl[unit], "Value High"=w171:dbl[unit], "dup VISA session"=w156:refnum<visa-resource-name>)  [unwired: 5 out]
        n198 = local write "Ch2High"(w171) -> ()
        n199 = local write "Ch2Low"(w170) -> ()
        n200 = call-dynamic "VISA Save Session.vi"("error in (no error)"=w155, "VISA Resource Name"=w156, "Instrument.lvclass in"=w159) -> ("error out"=w157:errorcluster, "Instrument.lvclass out"=w158:refnum<class "Pulse Generator.lvclass">)  [unwired: 7 out]
      }
      event "Modes (changes immediately)": Value Change {
        # "Don't need to populate member data in this screen because we trigger a read (which includes a check status)."
        n201 = event-data() -> ("NewVal"=w278:T2)  [unwired: 6 out]
        n202 = call-dynamic "VISA Get Session.vi"("error in (no error)"=w273, "Instrument.lvclass in"=w275) -> ("error out"=w272:errorcluster, "VISA Resource Name"=w274:refnum<visa-resource-name>, "Instrument.lvclass out"=w271:refnum<class "Pulse Generator.lvclass">)  [unwired: 7 out]
        n203 = property on="Read" class="Bool (strict)"("Val(Sgnl)"=TRUE ("Value (Signaling)")) -> ()  [unwired: 2 in, 2 out]
        n204 = property on="Enable/disable" class="Bool (strict)"("Val(Sgnl)"=TRUE ("Value (Signaling)")) -> ()  [unwired: 2 in, 2 out]
        n205 = case shown="\"Continuous Pulsed\", Default" w278 {
          tunnel: w274 -> [w282 w288 w292 w297 w301]
          tunnel: w272 -> [w281 w287 w291 w296 w300]
          tunnel: [w280 w286 w290 w295 w299] -> w268
          tunnel: [w279 w284 w289 w294 w298] -> w267
          frame "Continuous Pulsed", Default {
            n206 = call "HP81110A Generating Cont Pulses.vi"("error in (no error)"=w281, "Period Source (0:Internal)"=T3."Internal Oscillator", "VISA session"=w282) -> ("error out"=w280:errorcluster, "dup VISA session"=w279:refnum<visa-resource-name>)  [unwired: 1 in, 6 out]
          }
          frame "Continuous Pattern" {
            n207 = call "HP81110A Generating Cont Pattern.vi"("error in (no error)"=w287, "Period Source (0:Internal Oscillator)"=T4."Internal Oscillator", "VISA session"=w288) -> ("error out"=w286:errorcluster, "dup VISA session"=w284:refnum<visa-resource-name>)  [unwired: 1 in, 6 out]
          }
          frame "Internal Triggered Pattern" {
            n208 = call "HP81110A Generating Trigg Pattern.vi"("VISA session"=w292, "Trigger Source (0:Internal PLL)"=enum16{"Internal PLL", "External", "Manual"}."Internal PLL", "error in (no error)"=w291) -> ("dup VISA session"=w289:refnum<visa-resource-name>, "error out"=w290:errorcluster)  [unwired: 5 in, 6 out]
          }
          frame "External Triggered Pulsed" {
            n209 = call "HP81110A Generating Trigg Pulses.vi"("error in (no error)"=w296, "VISA session"=w297) -> ("error out"=w295:errorcluster, "dup VISA session"=w294:refnum<visa-resource-name>)  [unwired: 2 in, 6 out]
          }
          frame "External Triggered Pattern" {
            n210 = call "HP81110A Generating Trigg Pattern.vi"("VISA session"=w301, "Period Source (0:Internal Oscillator)"=T4."Internal Oscillator", "Trigger Source (0:Internal PLL)"=enum16{"Internal PLL", "External", "Manual"}."External", "error in (no error)"=w300) -> ("dup VISA session"=w298:refnum<visa-resource-name>, "error out"=w299:errorcluster)  [unwired: 4 in, 6 out]
          }
        }
        n211 = call-dynamic "VISA Save Session.vi"("error in (no error)"=w268, "VISA Resource Name"=w267, "Instrument.lvclass in"=w271) -> ("error out"=w269:errorcluster, "Instrument.lvclass out"=w270:refnum<class "Pulse Generator.lvclass">)  [unwired: 7 out]
      }
      event "Set Patterns": Value Change {
        # "Don't need to populate member data in this screen because we trigger a read (which includes a check status)."
        n212 = event-data() -> ()  [unwired: 7 out]
        n213 = local write "Set Patterns"(FALSE) -> ()
        n214 = property on="Read" class="Bool (strict)"("Val(Sgnl)"=TRUE ("Value (Signaling)")) -> ()  [unwired: 2 in, 2 out]
        n215 = local read "Strobe Pattern Set"() -> (w314:string)
        n216 = local read "Ch1Pattern Set"() -> (w316:string)
        n217 = local read "Ch2Pattern Set"() -> (w315:string)
        n218 = call "three string merge.vi"("Strobe String (def: 10)"=w314, "Ch2 String"=w315, "Ch1 String"=w316) -> ("Merged Output String"=w313:string)  [unwired: 8 out]
        n219 = call-dynamic "VISA Get Session.vi"("error in (no error)"=w311, "Instrument.lvclass in"=w312) -> ("error out"=w310:errorcluster, "VISA Resource Name"=w309:refnum<visa-resource-name>, "Instrument.lvclass out"=w308:refnum<class "Pulse Generator.lvclass">)  [unwired: 7 out]
        n220 = call "HP81110A Transfer String Into Memory.vi"("error in (no error)"=w310, "String"=w313, "Channel (1:Channel 1)"=T5."Channels Combined", "VISA session"=w309) -> ("error out"=w317:errorcluster, "dup VISA session"=w318:refnum<visa-resource-name>)  [unwired: 6 out]
        n221 = call "HP81110A Set Update Mode Of Pattern Data.vi"("error in (no error)"=w317, "Pattern Update Mode (1:Continuous)"=enum16{"Off", "Continuous", "Once"}."Once", "VISA session"=w318) -> ("error out"=w306:errorcluster, "dup VISA session"=w304:refnum<visa-resource-name>)  [unwired: 7 out]
        n222 = call-dynamic "VISA Save Session.vi"("error in (no error)"=w306, "VISA Resource Name"=w304, "Instrument.lvclass in"=w308) -> ("error out"=w305:errorcluster, "Instrument.lvclass out"=w307:refnum<class "Pulse Generator.lvclass">)  [unwired: 7 out]
      }
      event "Ch1 Toggle", "Ch1 NOT Toggle", "Ch2 Toggle", "Ch2 NOT Toggle", "Ch1/Ch2 Toggle": Value Change {
        n223 = event-data() -> ()  [unwired: 7 out]
        n224 = flat-sequence {
          tunnel: w327 -> [w330]
          tunnel: w328 -> [w331]
          tunnel: [w331] -> w324
          tunnel: [w330] -> w323
          tunnel: [w350] -> w326
          tunnel: [w341] -> w325
          tunnel: w324 -> [w353]
          tunnel: w323 -> [w352]
          frame #0 {
            n225 = local read "Ch1/Ch2 Toggle"() -> (w329:bool)
            n226 = case shown="True" w329 {
              frame False {
              }
              frame True {
                n227 = local read "Ch1 Toggle"() -> (w334:bool)
                n228 = local read "Ch2 Toggle"() -> (w333:bool)
                n229 = Not(x=w334) -> (.not. x?=w335:bool)
                n230 = Not(x=w333) -> (.not. x?=w332:bool)
                n231 = local write "Ch1 Toggle"(w335) -> ()
                n232 = local write "Ch2 Toggle"(w332) -> ()
              }
            }
          }
          frame #1 {
            n233 = local read "Ch1 NOT Toggle"() -> (w348:bool)
            n234 = local read "Ch2 NOT Toggle"() -> (w347:bool)
            n235 = local read "Ch1 Toggle"() -> (w339:bool)
            n236 = local read "Ch2 Toggle"() -> (w337:bool)
            n237 = local read "Ch1 Sync"() -> (w354:bool)
            n238 = local read "Ch2 Sync"() -> (w349:bool)
            n239 = case shown="True" w354 {
              tunnel: [w357 w358] -> w338
              tunnel: w348 -> [w357 _]
              tunnel: w339 -> [_ w358]
              frame False {
              }
              frame True {
                n240 = local write "Ch1 NOT Toggle"(w358) -> ()
              }
            }
            n241 = case shown="True" w349 {
              tunnel: [w355 w356] -> w336
              tunnel: w347 -> [w355 _]
              tunnel: w337 -> [_ w356]
              frame False {
              }
              frame True {
                n242 = local write "Ch2 NOT Toggle"(w356) -> ()
              }
            }
            n243 = call-dynamic "VISA Get Session.vi"("error in (no error)"=w352, "Instrument.lvclass in"=w353) -> ("error out"=w345:errorcluster, "VISA Resource Name"=w346:refnum<visa-resource-name>, "Instrument.lvclass out"=w351:refnum<class "Pulse Generator.lvclass">)  [unwired: 7 out]
            n244 = call "HP81110A Output Set - Fast.vi"("notoutput2"=w336, "output1"=w339, "error in (no error)"=w345, "output2"=w337, "notoutput1"=w338, "VISA session"=w346) -> ("error out"=w343:errorcluster, "dup VISA session"=w344:refnum<visa-resource-name>)  [unwired: 4 out]
            n245 = Build Array(w339, w338, w337, w336) -> (w340:bool[])
            n246 = call-dynamic "VISA Save Session.vi"("error in (no error)"=w343, "VISA Resource Name"=w344, "Instrument.lvclass in"=w351) -> ("error out"=w350:errorcluster, "Instrument.lvclass out"=w342:refnum<class "Pulse Generator.lvclass">)  [unwired: 7 out]
            n247 = Bundle By Name(cluster=w342, "Outputs 1/!1/2/!2"=w340) -> (w341:refnum<class "Pulse Generator.lvclass">)
          }
        }
      }
      event "OverallPeriodSet": Value Change {
        n248 = event-data() -> ("NewVal"=w359:dbl[unit])  [unwired: 6 out]
        n249 = Reciprocal(x=w359) -> (1/x=w364:dbl[unit])
        n250 = local write "OverallFreqSet"(w364) -> ()
        n251 = local read "Width/Duty\nUP/DOWN Ch1"() -> (w361:bool)
        n252 = local read "Width/Duty\nUP/DOWN Ch2"() -> (w360:bool)
        n253 = case shown="True" w361 {
          tunnel: w359 -> [w377 w380]
          frame False {
            n254 = local read "Ch1Duty (%) Set"() -> (w375:dbl)
            n255 = Divide(x=w375, y=100.0) -> (x/y=w378:dbl)
            n256 = Multiply(x=w378, y=w377) -> (x*y=w376:dbl[unit])
            n257 = local write "Ch1Width"(w376) -> ()
          }
          frame True {
            n258 = local read "Ch1Width"() -> (w381:dbl[unit])
            n259 = Divide(x=w381, y=w380) -> (x/y=w384:dbl)
            n260 = Multiply(x=w384, y=100) -> (x*y=w383:dbl)
            n261 = local write "Ch1Duty (%) Set"(w383) -> ()
          }
        }
        n262 = case shown="True" w360 {
          tunnel: w359 -> [w366 w374]
          frame False {
            n263 = local read "Ch2Duty (%) Set"() -> (w369:dbl)
            n264 = Divide(x=w369, y=100.0) -> (x/y=w368:dbl)
            n265 = Multiply(x=w368, y=w366) -> (x*y=w365:dbl[unit])
            n266 = local write "Ch2Width"(w365) -> ()
          }
          frame True {
            n267 = local read "Ch2Width"() -> (w373:dbl[unit])
            n268 = Divide(x=w373, y=w374) -> (x/y=w372:dbl)
            n269 = Multiply(x=w372, y=100) -> (x*y=w370:dbl)
            n270 = local write "Ch2Duty (%) Set"(w370) -> ()
          }
        }
      }
      event "OverallFreqSet": Value Change {
        n271 = event-data() -> ("NewVal"=w396:dbl[unit])  [unwired: 6 out]
        n272 = local read "Ch1Width"() -> (w395:dbl[unit])
        n273 = local read "Ch2Width"() -> (w394:dbl[unit])
        n274 = Reciprocal(x=w396) -> (1/x=w393:dbl[unit])
        n275 = local write "OverallPeriodSet"(w393) -> ()
        n276 = Divide(x=w395, y=w393) -> (x/y=w390:dbl)
        n277 = Divide(x=w394, y=w393) -> (x/y=w388:dbl)
        n278 = Multiply(x=w390, y=100) -> (x*y=w389:dbl)
        n279 = Multiply(x=w388, y=100) -> (x*y=w387:dbl)
        n280 = local write "Ch1Duty (%) Set"(w389) -> ()
        n281 = local write "Ch2Duty (%) Set"(w387) -> ()
      }
      event "stop": Value Change {
        n282 = event-data() -> ()  [unwired: 7 out]
      }
      event "Width/Duty\nUP/DOWN Ch1", "Width/Duty\nUP/DOWN Ch2": Value Change {
        n283 = event-data() -> ()  [unwired: 7 out]
        n284 = local read "Width/Duty\nUP/DOWN Ch2"() -> (w408:bool)
        n285 = local read "Width/Duty\nUP/DOWN Ch1"() -> (w409:bool)
        n286 = Select(t=2, s=w408, f=0) -> (s? t:f=w401:i32)
        n287 = Select(t=2, s=w409, f=0) -> (s? t:f=w400:i32)
        n288 = property on="Ch2Duty (%) Set" class="DigNum (strict)"("Disabled"=w401) -> ()  [unwired: 2 in, 2 out]
        n289 = property on="Ch2Duty (%)" class="DigNum (strict)"("Disabled"=w401) -> ()  [unwired: 2 in, 2 out]
        n290 = property on="Ch1Duty (%) Set" class="DigNum (strict)"("Disabled"=w400) -> ()  [unwired: 2 in, 2 out]
        n291 = property on="Ch1Duty (%)" class="DigNum (strict)"("Disabled"=w400) -> ()  [unwired: 2 in, 2 out]
        n292 = local read "Width/Duty\nUP/DOWN Ch1"() -> (w407:bool)
        n293 = local read "Width/Duty\nUP/DOWN Ch2"() -> (w406:bool)
        n294 = Select(t=0, s=w407, f=2) -> (s? t:f=w403:i32)
        n295 = Select(t=0, s=w406, f=2) -> (s? t:f=w402:i32)
        n296 = property on="Ch1Width" class="DigNum (strict)"("DisabledEnum"=w403) -> ()  [unwired: 2 in, 2 out]
        n297 = property on="Ch2Width" class="DigNum (strict)"("DisabledEnum"=w402) -> ()  [unwired: 2 in, 2 out]
        n298 = property on="Ch1WidthSet" class="DigNum (strict)"("DisabledEnum"=w403) -> ()  [unwired: 2 in, 2 out]
        n299 = property on="Ch2WidthSet" class="DigNum (strict)"("DisabledEnum"=w402) -> ()  [unwired: 2 in, 2 out]
        n300 = Bundle By Name(cluster=w405, "Ch1Width(true)"=w407, "Ch2Width(true)"=w406) -> (w404:refnum<class "Pulse Generator.lvclass">)
      }
      event "Ch1Duty (%) Set": Value Change {
        # "this hard codes to have the duty cycle be read as a width"
        n301 = event-data() -> ()  [unwired: 7 out]
        n302 = local read "Ch1WidthSet"() -> (w423:dbl[unit])
        n303 = local read "Ch1Duty (%) Set"() -> (w427:dbl)
        n304 = local read "OverallPeriodSet"() -> (w425:dbl[unit])
        n305 = local read "Width/Duty\nUP/DOWN Ch1"() -> (w422:bool)
        n306 = Divide(x=w427, y=100.0) -> (x/y=w426:dbl)
        n307 = Multiply(x=w426, y=w425) -> (x*y=w424:dbl[unit])
        n308 = Select(t=w423, s=w422, f=w424) -> (s? t:f=w421:dbl[unit])
        n309 = local write "Ch1WidthSet"(w421) -> ()
      }
      event "Ch2Duty (%) Set": Value Change {
        # "this hard codes to have the duty cycle be read as a width"
        n310 = event-data() -> ()  [unwired: 7 out]
        n311 = local read "Ch2WidthSet"() -> (w432:dbl[unit])
        n312 = local read "Ch2Duty (%) Set"() -> (w438:dbl)
        n313 = local read "OverallPeriodSet"() -> (w435:dbl[unit])
        n314 = local read "Width/Duty\nUP/DOWN Ch2"() -> (w433:bool)
        n315 = Divide(x=w438, y=100.0) -> (x/y=w436:dbl)
        n316 = Multiply(x=w436, y=w435) -> (x*y=w434:dbl[unit])
        n317 = Select(t=w432, s=w433, f=w434) -> (s? t:f=w431:dbl[unit])
        n318 = local write "Ch2WidthSet"(w431) -> ()
      }
      event "Ch1WidthSet": Value Change {
        n319 = event-data() -> ("NewVal"=w445:dbl[unit])  [unwired: 6 out]
        n320 = local read "OverallPeriodSet"() -> (w444:dbl[unit])
        n321 = Divide(x=w445, y=w444) -> (x/y=w443:dbl)
        n322 = Multiply(x=100, y=w443) -> (x*y=w441:dbl)
        n323 = local write "Ch1Duty (%) Set"(w441) -> ()
      }
      event "Ch2WidthSet": Value Change {
        n324 = event-data() -> ("NewVal"=w448:dbl[unit])  [unwired: 6 out]
        n325 = local read "OverallPeriodSet"() -> (w452:dbl[unit])
        n326 = Divide(x=w448, y=w452) -> (x/y=w451:dbl)
        n327 = Multiply(x=100, y=w451) -> (x*y=w449:dbl)
        n328 = local write "Ch2Duty (%) Set"(w449) -> ()
      }
    }
    n329 = call-dynamic "VISA Get Session.vi"("error in (no error)"=w30, "Instrument.lvclass in"=w31) -> ("error out"=w29:errorcluster, "VISA Resource Name"=w35:refnum<visa-resource-name>, "Instrument.lvclass out"=w33:refnum<class "Pulse Generator.lvclass">)  [unwired: 7 out]
    n330 = call "HP81110A Error Query.vi"("VISA session"=w35, "error in (no error)"=w29) -> ("dup VISA session"=w34:refnum<visa-resource-name>, "error out"=w38:errorcluster)  [unwired: 12 out]
    n331 = call <vilib>:"Simple Error Handler.vi"("error in (no error)"=w38) -> ("error out"=w28:errorcluster)  [unwired: 1 in, 7 out]
    n332 = call-dynamic "VISA Save Session.vi"("error in (no error)"=w28, "VISA Resource Name"=w34, "Instrument.lvclass in"=w33) -> ("error out"=w27:errorcluster, "Instrument.lvclass out"=w32:refnum<class "Pulse Generator.lvclass">)  [unwired: 7 out]
  }
  n333 = call-dynamic "_Destroy.vi"("error in (no error)"=w15, "Instrument in"=w16) -> ("error out"=→"error out":errorcluster)  [unwired: 9 out]
